vi "Open Poly VI Ref.vi"(8 "error in":errorcluster, 11 "Poly VI Path":path) -> (0 "error out":errorcluster, 1 "Status":string, 2 "Name":string, 3 "Refnum out":refnum<vi>, 5 "Success?":bool)   [LabVIEW 2020, in "Data Type Scripting.lvlib"]
uses:
  Data Type Scripting.lvlib
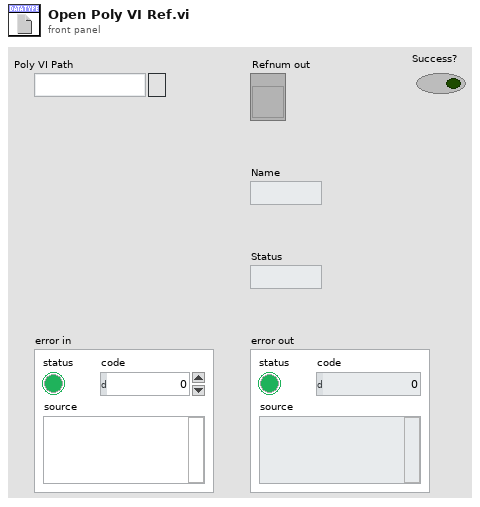
[diagram p1: front panel]
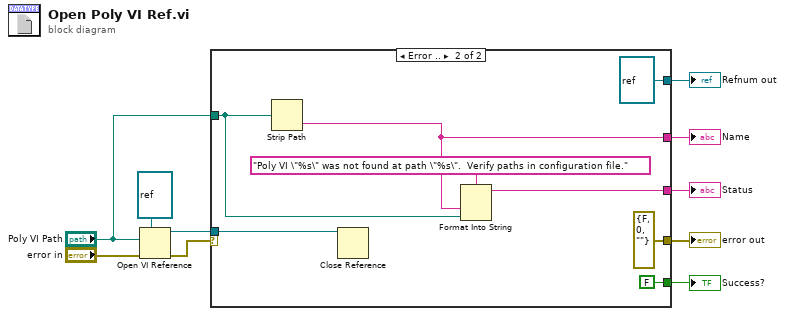
[diagram p0: block diagram]
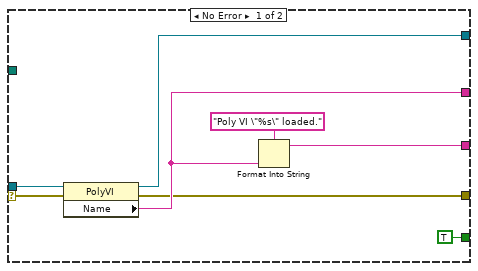
[diagram p2: hidden frame]
diagram:
  n1 = Open VI Reference(type specifier VI Refnum (for type only)=refnum<vi> refnum, vi path="Poly VI Path", error in (no error)="error in") -> (vi reference=w6:refnum<vi>, error out=w4:errorcluster)  [unwired: 3 in]
  n2 = case shown="Error .." w4 {
    selector: w4 -> [w12 _]
    tunnel: [w18 refnum<vi> refnum ("type specifier VI Refnum (for type only)")] -> w10
    tunnel: [w16 w23] -> w9
    tunnel: [w15 w25] -> w8
    tunnel: [w14 errorcluster {"status"=FALSE, "code"=0, "source"=""} ("error out")] -> w7
    tunnel: w6 -> [w13 w22]
    tunnel: "Poly VI Path" -> [_ w24]
    tunnel: [TRUE FALSE] -> w1
    frame No Error {
      n3 = property class="PolyVI"(reference=w13, error in=w12) -> (reference out=w18:refnum<vi>, error out=w14:errorcluster, "Name"=w16:string)
      n4 = Format Into String(format string="Poly VI \"%s\" loaded.", w16) -> (resulting string=w15:string)  [unwired: 2 in, 1 out]
    }
    frame Error {
      n5 = Strip Path(path=w24) -> (name=w23:string)  [unwired: 1 out]
      n6 = Close Reference(reference=w22) -> ()  [unwired: 1 in, 1 out]
      n7 = Format Into String(format string="Poly VI \"%s\" was not found at path \"%s\".  Verify paths in configuration file.", w23, w24) -> (resulting string=w25:string)  [unwired: 2 in, 1 out]
    }
  }
  "Refnum out" <- w10
  "Name" <- w9
  "Status" <- w8
  "error out" <- w7
  "Success?" <- w1
